vi "SA5G_getEVM_Only.vi"(8 "error in":errorcluster, 11 "VISA in":refnum<visa-resource-name>) -> (0 "error out":errorcluster, 1 "All":dbl[](array[numeric]) format="%#.3g", 2 "get_EVM":T1, 3 "VISA out":refnum<visa-resource-name>)   [LabVIEW 2020, in "Keysight.lvlib"]
uses:
  Keysight.lvlib
panel:
  out "Response":string
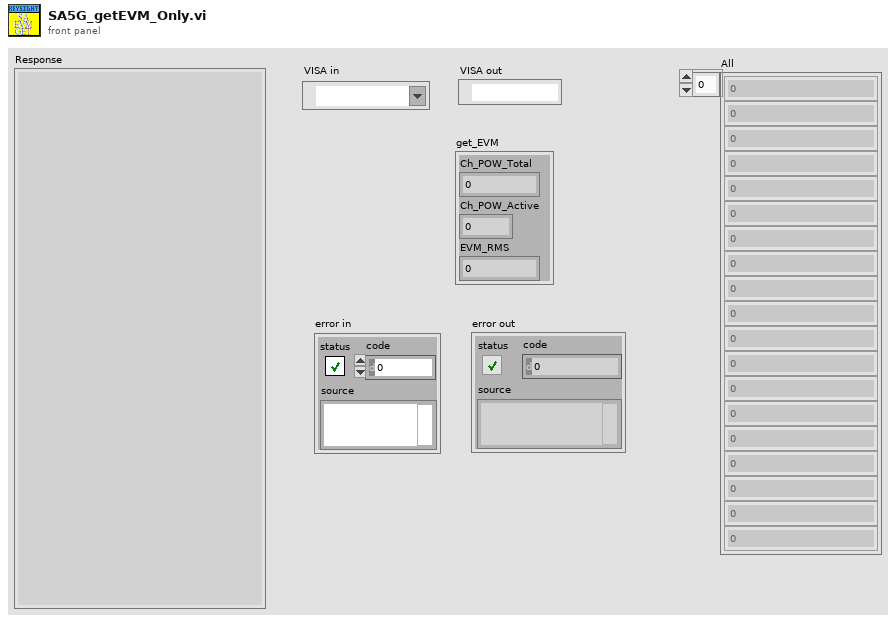
[diagram p1: front panel]
types:
  T1 = cluster{"Ch_POW_Total":dbl, "Ch_POW_Active":dbl, "EVM_RMS":dbl}
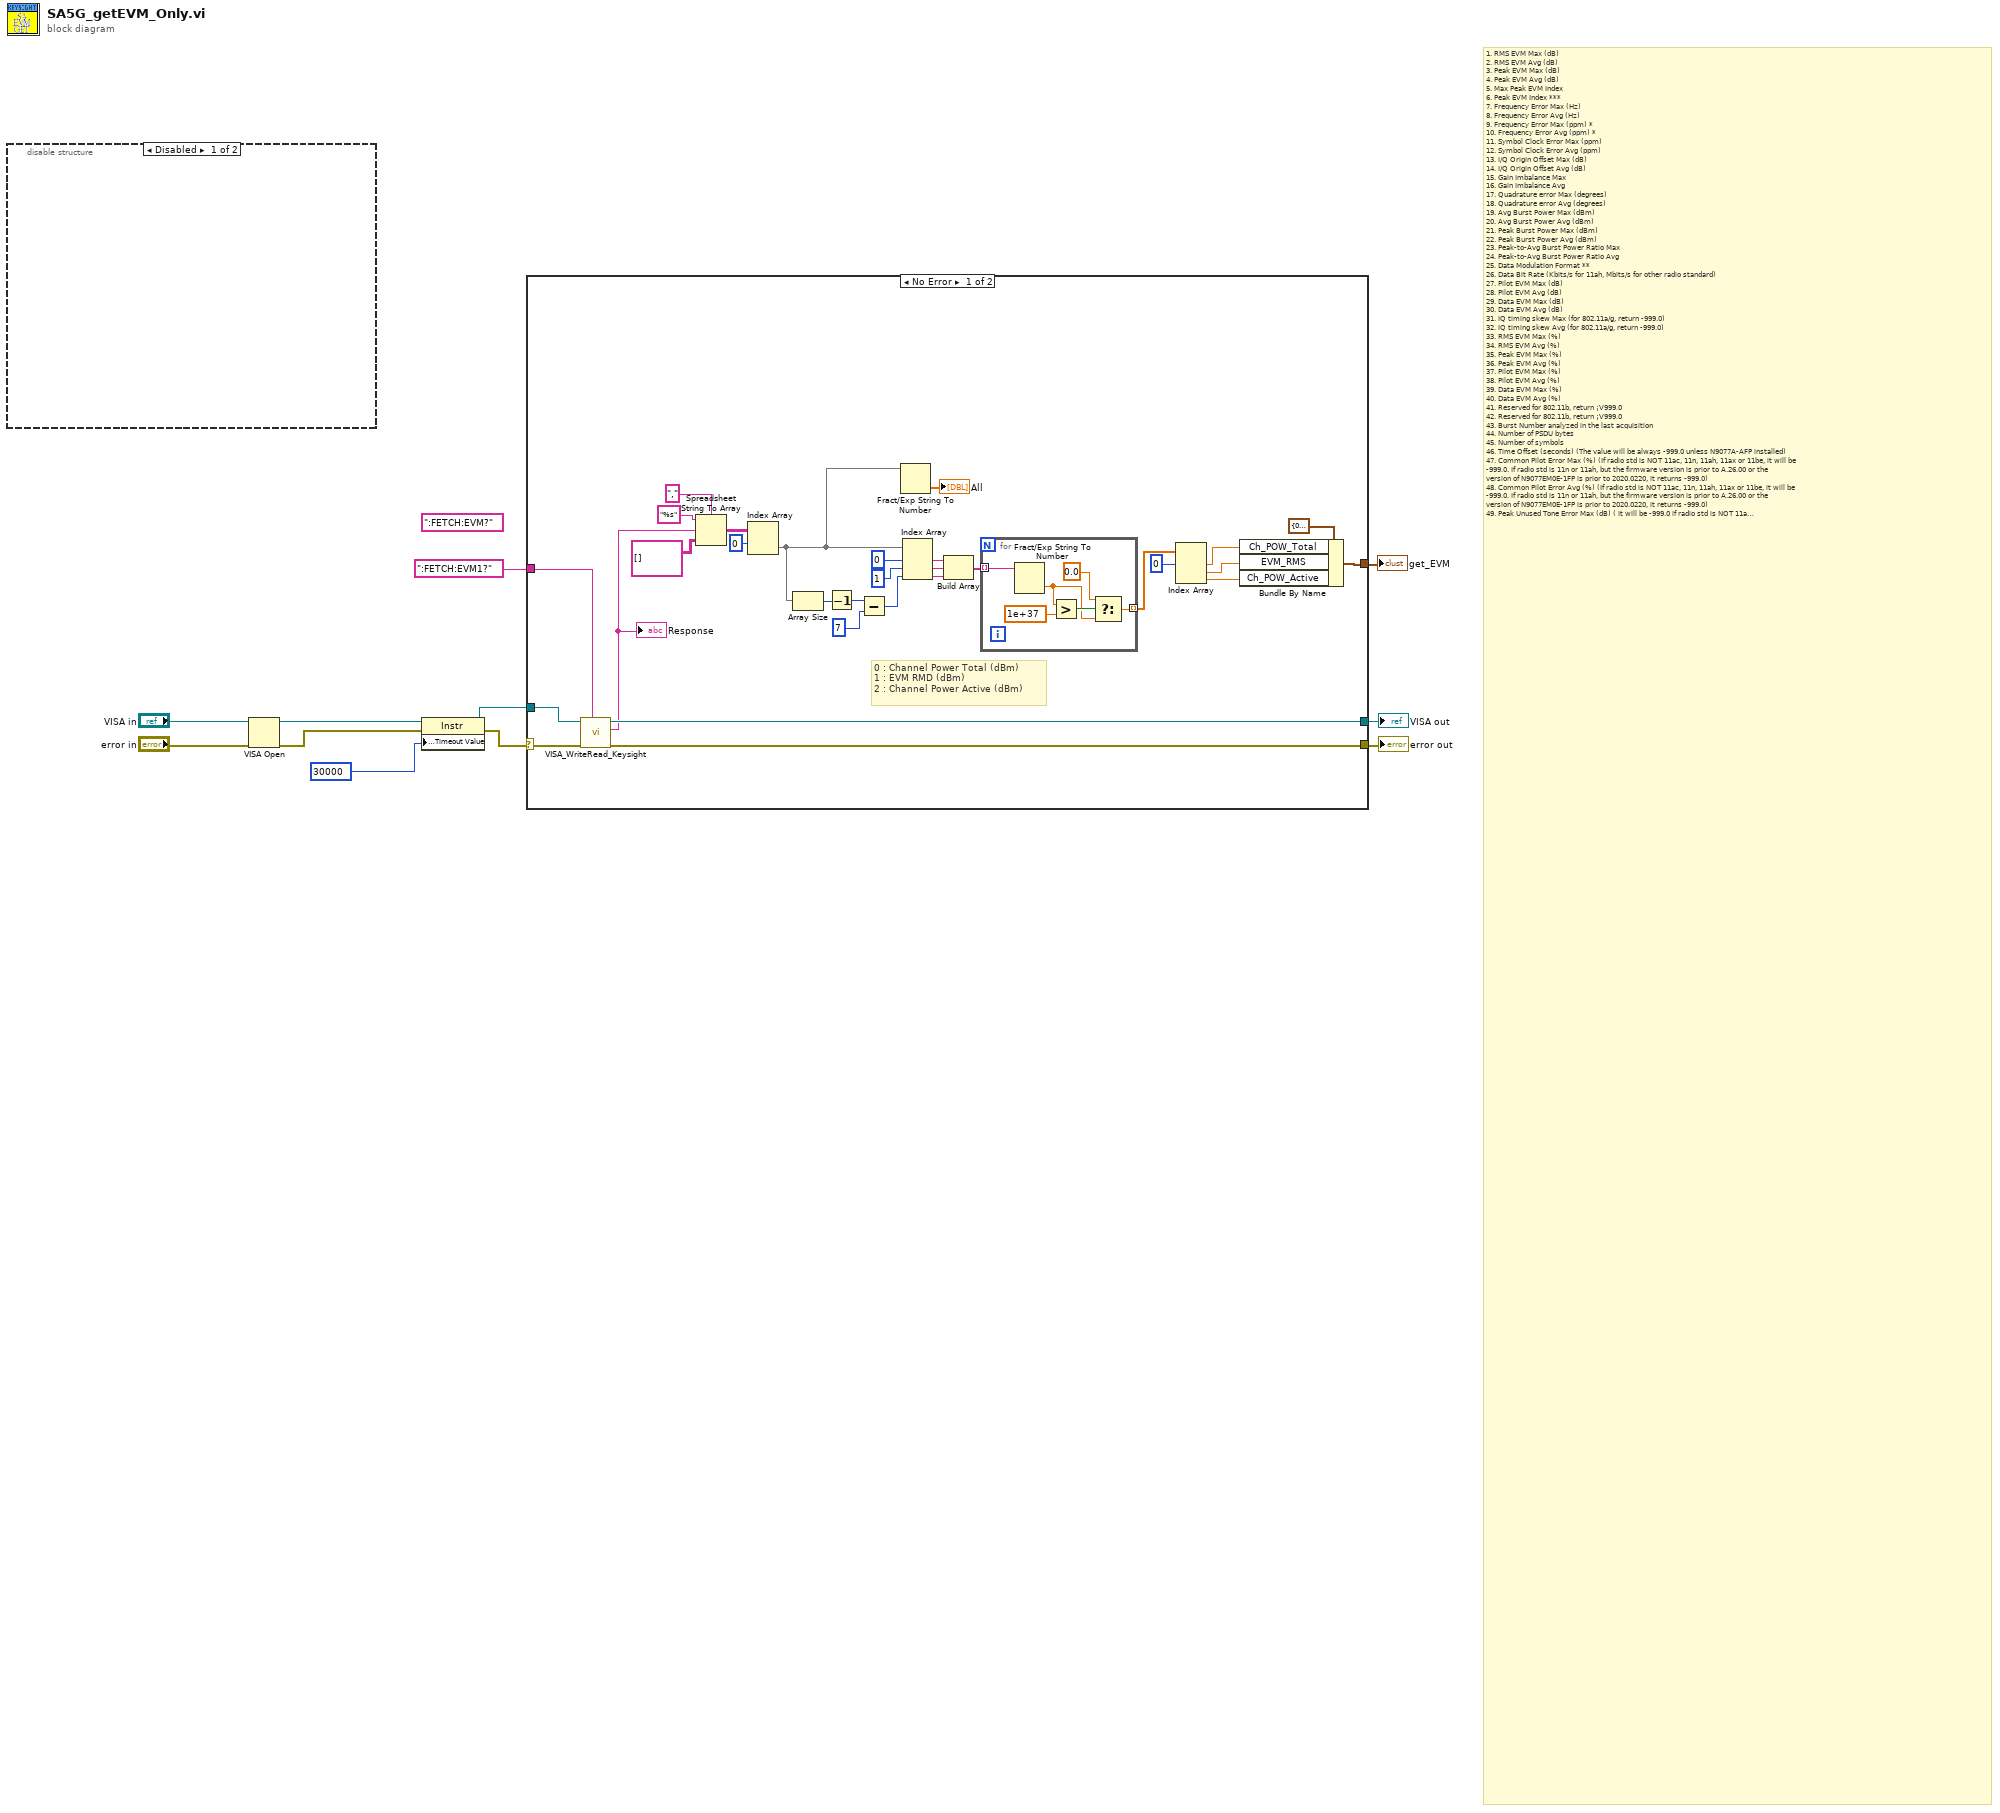
[diagram p0: block diagram]
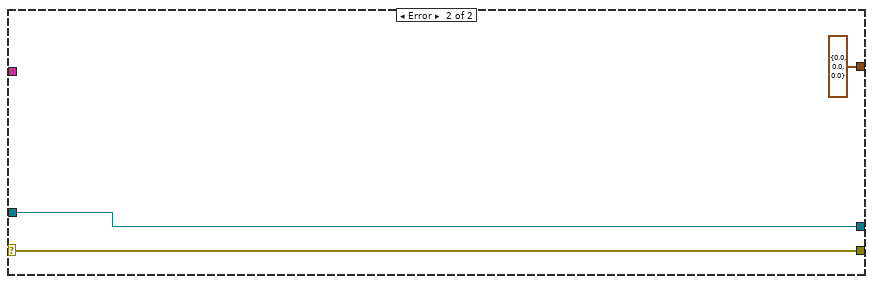
[diagram p3: hidden frame]
diagram:
  (unwired) ":FETCH:EVM?" ("write buffer")
  # "1. RMS EVM Max (dB)\n2. RMS EVM Avg (dB)\n3. Peak EVM Max (dB)\n4. Peak EVM Avg (dB)\n5. Max Peak EVM Index\n6. Peak EVM Index ***\n7. Frequency Error Max (Hz)\n8. Frequency Error Avg (Hz)\n9. Frequency Error Max (ppm) *\n10. Frequency Error Avg (ppm) *\n11. Symbol Clock Error Max (ppm)\n12. Symbol Clock Error Avg (ppm)\n13. I/Q Origin Offset Max (dB)\n14. I/Q Origin Offset Avg (dB)\n15. Gain Imbalance Max\n16. Gain Imbalance Avg\n17. Quadrature error Max (degrees)\n18. Quadrature error Avg (degrees)\n19. Avg Burst Power Max (dBm)\n20. Avg Burst Power Avg (dBm)\n21. Peak Burst Power Max (dBm)\n22. Peak Burst Power Avg (dBm)\n23. Peak-to-Avg Burst Power Ratio Max\n24. Peak-to-Avg Burst Power Ratio Avg\n25. Data Modulation Format **\n26. Data Bit Rate (Kbits/s for 11ah, Mbits/s for other radio standard)\n27. Pilot EVM Max (dB)\n28. Pilot EVM Avg (dB)\n29. Data EVM Max (dB)\n30. Data EVM Avg (dB)\n31. IQ timing skew Max (for 802.11a/g, return -999.0)\n32. IQ timing skew Avg (for 802.11a/g, return -999.0)\n33. RMS EVM Max (%)\n34. RMS EVM Avg (%)\n35. Peak EVM Max (%)\n36. Peak EVM Avg (%)\n37. Pilot EVM Max (%)\n38. Pilot EVM Avg (%)\n39. Data EVM Max (%)\n40. Data EVM Avg (%)\n41. Reserved for 802.11b, return ¡V999.0\n42. Reserved for 802.11b, return ¡V999.0\n43. Burst Number analyzed in the last acquisition\n44. Number of PSDU bytes\n45. Number of symbols\n46. Time Offset (seconds) (The value will be always -999.0 unless N9077A-AFP installed)\n47. Common Pilot Error Max (%) (If radio std is NOT 11ac, 11n, 11ah, 11ax or 11be, it will be\n-999.0. If radio std is 11n or 11ah, but the firmware version is prior to A.26.00 or the\nversion of N9077EM0E-1FP is prior to 2020.0220, it returns -999.0)\n48. Common Pilot Error Avg (%) (If radio std is NOT 11ac, 11n, 11ah, 11ax or 11be, it will be\n-999.0. If radio std is 11n or 11ah, but the firmware version is prior to A.26.00 or the\nversion of N9077EM0E-1FP is prior to 2020.0220, it returns -999.0)\n49. Peak Unused Tone Error Max (dB) ( It will be -999.0 if radio std is NOT 11ax or 11be)\n50. Peak Unused Tone Error Avg (dB) ( It will be -999.0 if radio std is NOT 11ax or 11be)\n51. Symbol Index for Peak Unused Tone Error Max ( It will be -999.0 if radio std is NOT 11ax\nor 11be)\n52. Ru Index for Peak Unused Tone Error Max ( It will be -999.0 if radio std is NOT 11ax or\n11be)\n53. HE/EHT PPDU type ( it is 0~6 and will always be -999 if radio std is NOT 11ax or 11be)\nFor the 53rd result, HE/EHT PPDU type, the returned integer means:\n0 HE_SU\n1 HE_MU\n2 HE_Extended Range SU\n3 HE_TriggerBased\n4 HE_SU_Sounding_NDP\n5 HE_TriggerBased_NDP\n6 EHT_MU\n7 EHT_TriggerBased\n8 EHT_Sounding_NDP\n-999 Unknown\n54. Common Pilot Error Max (Degree) (If radio std is NOT 11ac, 11n, 11ah, 11ax or 11be, it\nwill be -999.0. If radio std is 11n or 11ah, but the firmware version is prior to A.26.00 or\nthe version of N9077EM0E-1FP is prior to 2020.0220, it returns -999.0)\n55. Common Pilot Error Avg (Degree) (If radio std is NOT 11ac, 11n, 11ah, 11ax or 11be, it\nwill be -999.0. If radio std is 11n or 11ah, but the firmware version is prior to A.26.00 or\nthe version of N9077EM0E-1FP is prior to 2020.0220, it returns -999.0)\n56. Packet Extension Duration (us) ( it will be -999.0 if radio std is NOT 11ax or 11be)\n57. Guard Interval of Trigger-based PPDU Guard Interval (us) ( it will be -999.0 if radio std is\nNOT 11ax or 11be)\n58. HE-LTF/EHT-LTF type of Trigger-based PPDU if radio std is 11ax/11be; it will be -999.0\nif radio std is NOT 11ax or 11be\nHE-LTF Type of Trigger-based PPDU, the returned integer means:\n0 1 x LTF\n1 2 x LTF\n2 4 x LTF\nEHT-LTF Type of Trigger-based PPDU, the returned integer means:\n1 2 x LTF\n2 4 x LTF\n59. The minimal Meas Interval for successful PSDU CRC decoding (if the Firmware Version\nis below A.22.00, it returns -999.0 which means Invalid)\n60. PSDU CRC for 802.11a/11n/11ac/11af (if the Firmware Version is below A.22.00 or it is\nnot 802.11a/11n/11ac/11af , 1 means Fail, 0 means Pass, -999 means Invalid)\n61. Duty On Period (Unit is microseconds, it is the pulse width, if the Firmware Version is\nbelow A.30.00 or it is not found, it returns -999.0 which means Invalid.-999.0 means\ninvalid)\n62. Duty Off Period (Unit is microseconds, it is (pulse period ¡V pulse width), if the Firmware\nVersion is below A.30.00 or it is not found, it returns -999.0 which means Invalid.)\n63. Duty Cycle (Unit is %, it is pulse width / pulse period, if the Firmware Version is below\nA.30.00 or (either Duty On or Off is not found), it returns -999.0 which means Invalid\n64. Average RMS ccEVM, if the Firmware Version is below A.33.00 or Cross-Correlated\nEVM is off, it returns -999.0 which means Invalid.\nHere ¡§Average¡¨ means using data of each measurement in measurement loop to\ncalculate RMS ccEVM.\nccEVM is not accurate and can¡¦t reflect source EVM if data point is not sufficient, use\nmore data points (average number * Data Points), then it can lead to a more stable and\naccurate ccEVM result.\nIt will not only benefit for the cases that data point is obviously not sufficient (small BW,\nsmall MCS, small symbol length), for all cases, it will lead to a more accurate ccEVM\nresult, the key point is to balance time and improvement\n65. Valid data points that used to calculate ccEVM, if the Firmware Version is below A.33.00\nor ccEVM is off, it returns -999.0 which means Invalid\n66. Total data points that used to calculate ccEVM, if the Firmware Version is below A.33.00\nor ccEVM is off, it returns -999.0 which means Invalid\n67. Partial Burst Power Max (dBm), if the Firmware Version is below A.36 Minor or Radio Std\nis not 11n/ac/ax/be, returns -999.0, which means Invalid. Valid when Radio Std is 11agjp\nif Radio Std Detection is auto, but invalid if Radio Std Detection is Manual\n68. Partial Burst Power Avg(dBm) if the Firmware Version is below A.36 Minor or Radio Std\nis not 11n/ac/ax/be, returns -999.0, which means Invalid. Valid when Radio Std is 11agjp\nif Radio Std Detection is auto, but invalid if Radio Std Detection is Manual"
  n1 = disable-structure shown="Disabled" {
    frame Disabled {
    }
    frame Enabled {
    }
  }
  n2 = VISA Open(error in (no error)="error in", VISA resource name="VISA in") -> (VISA resource name=w2:refnum<visa-resource-name>, error out=w4:errorcluster)  [unwired: 3 in]
  n3 = property on="Property Node" class="Instr"(reference=w2, error in=w4, "General Settings:Timeout Value"=u32 30000) -> (reference out=w6:refnum<visa-resource-name>, error out=w7:errorcluster)
  n4 = case shown="No Error" w7 {
    selector: w7 -> [w37 w50]
    tunnel: [w41 w50] -> w10
    tunnel: [w40 w49] -> w11
    tunnel: ":FETCH:EVM1?" ("write buffer") -> [w39 _]
    tunnel: w6 -> [w38 w49]
    tunnel: [w15 T1 {"Ch_POW_Total"=0.0, "Ch_POW_Active"=0.0, "EVM_RMS"=0.0} ("get_EVM")] -> w5
    frame No Error {
      # "0 : Channel Power Total (dBm)\n1 : EVM RMD (dBm)\n2 : Channel Power Active (dBm)"
      n5 = call "VISA_WriteRead_Keysight.vi"("VISA_CMD"=w39, "error in"=w37, "VISA in"=w38) -> ("error out"=w41:errorcluster, "Response"=w31:string, "VISA out"=w40:refnum<visa-resource-name>)  [unwired: 6 in]
      "Response" <- w31
      n6 = Spreadsheet String To Array(delimiter (Tab)="," ("format string"), format string="%s", spreadsheet string=w31, array type (2D Dbl)=string[][] [] ("Array")) -> (array=w36:string[][])
      n7 = Index Array(array=w36, index (row)=0) -> (element=w13:string[])  [unwired: 1 in]
      n8 = Array Size(array=w13) -> (size(s)=w30:i32)
      n9 = Decrement(x=w30) -> (x-1=w29:i32)
      n10 = Subtract(x=w29, y=7) -> (x-y=w25:i32)
      n11 = Fract/Exp String To Number(string=w13) -> (number=→"All":dbl[])  [unwired: 3 in, 1 out]
      n12 = Index Array(array=w13, index #1=0 ("index"), index #2=1 ("index"), index #3=w25) -> (element #1=w14:string, element #2=w24:string, element #3=w23:string)
      n13 = Build Array(w14, w24, w23) -> (w22:string[])
      n14 = for {
        tunnel: w22 -> [w43] mode=indexing
        tunnel: [w42] -> w20 mode=indexing
        n15 = Fract/Exp String To Number(string=w43) -> (number=w45:dbl)  [unwired: 3 in, 1 out]
        n16 = Greater?(x=w45, y=1e+37 ("number")) -> (0:w46:bool)
        n17 = Select(t=0.0, s=w46, f=w45) -> (s? t:f=w42:dbl)
      }
      n18 = Index Array(array=w20, index #1=0 ("index")) -> (element #1=w18:dbl, element #2=w17:dbl, element #3=w16:dbl)  [unwired: 2 in]
      n19 = Bundle By Name(cluster=T1 {"Ch_POW_Total"=0.0, "Ch_POW_Active"=0.0, "EVM_RMS"=0.0} ("get_EVM"), "Ch_POW_Total"=w18, "EVM_RMS"=w17, "Ch_POW_Active"=w16) -> (w15:T1)
    }
    frame Error {
    }
  }
  "VISA out" <- w11
  "error out" <- w10
  "get_EVM" <- w5
